vi "Query with OPC sync.vi"(7 "Timeout (0 = OPC timeout)":i32, 8 "error in (no error)":errorcluster, 10 "Query":string, 11 "VISA resource name":refnum<visa-resource-name>) -> (0 "error out":errorcluster, 2 "Response Value":string, 3 "VISA resource name out":refnum<visa-resource-name>)   [LabVIEW 2015, in "Rohde&Schwarz CMP LR WPAN Measurement.lvlib"]
doc: "This VI sends SCPI query to the instrument synchronised with OPC-polling. Use this function to wait for a response that can take a long time to complete e.g. self-alignment, calibration or self-test."
uses:
  <instrlib>/Rohde&Schwarz CMP LR WPAN Measurement/Rohde&Schwarz CMP LR WPAN Measurement.lvlib
  <instrlib>/Rohde&Schwarz CMP LR WPAN Measurement/Private/rsidr_core.llb/rsidr_core.lvlib
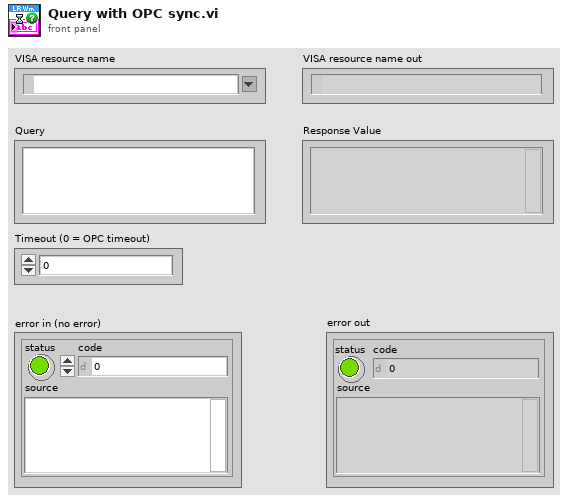
[diagram p1: front panel]
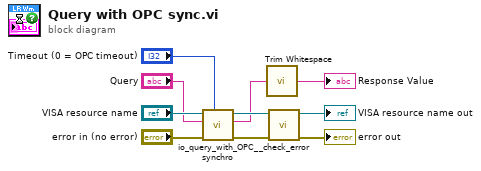
[diagram p0: block diagram]
diagram:
  n1 = call <instrlib>:"io_query_with_OPC_synchro.vi"("Timeout in (0 = OPC timeout)"="Timeout (0 = OPC timeout)", "error in"="error in (no error)", "write buffer"="Query", "VISA resource name"="VISA resource name") -> ("error out"=w8:errorcluster, "read buffer"=w1:string, "VISA resource name out"=w7:refnum<visa-resource-name>)  [unwired: 5 in]
  n2 = call <vilib>:"Trim Whitespace.vi"("string"=w1) -> ("trimmed string"=→"Response Value":string)  [unwired: 1 in]
  n3 = call <instrlib>:"_check_error.vi"("error in (no error)"=w8, "VISA resource name"=w7) -> ("error out"=→"error out":errorcluster, "VISA resource name out"=→"VISA resource name out":refnum<visa-resource-name>)  [unwired: 8 in]
